vi "Enqueue.vi"(5 "QueName":string="BaseVisQue", 7 "Priority? (F)":bool, 8 "Error":errorcluster[](array[cluster]), 9 "Data":variant, 10 "Message":string) -> (0 "Error":errorcluster[](array[cluster]))   [LabVIEW 2017, in "Visualization.lvlib" / "VisualizeBase_class.lvclass"]
uses:
  VisializeBase_class/VisualizeBase_class.lvclass
  Typedefs/MsgType.ctl
  <userlib>/NIST/NISTErrorLib/NISTErrorLib.lvlib
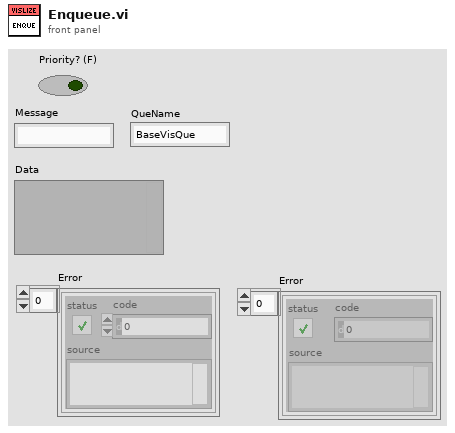
[diagram p1: front panel]
types:
  T1 = typedef "Visualization.lvlib/VisualizeBase_class.lvclass/MsgType.ctl" = cluster{"Message":string, "Data":variant}
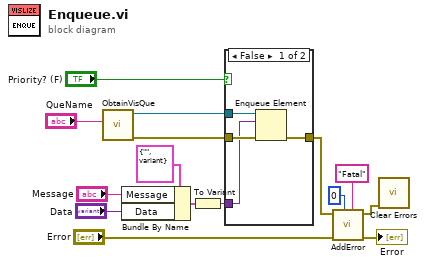
[diagram p0: block diagram]
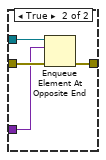
[diagram p2: hidden frame]
diagram:
  n1 = call "ObtainVisQue.vi"("QueName"="QueName") -> ("error out"=w10:errorcluster, "queue out"=w14:refnum<queue>)  [unwired: 9 in]
  n2 = Bundle By Name(cluster=T1 {"Message"="", "Data"=variant} ("clMsgType"), "Message"="Message", "Data"="Data") -> (w9:T1)
  n3 = To Variant(anything=w9) -> (Variant=w8:variant)
  n4 = case shown="False" "Priority? (F)" {
    tunnel: w14 -> [w18 w23]
    tunnel: w10 -> [w19 w22]
    tunnel: w8 -> [w17 w21]
    tunnel: [w16 w20] -> w7
    frame False {
      n5 = Enqueue Element(queue=w18, element=w17, error in (no error)=w19) -> (error out=w16:errorcluster)  [unwired: 1 in, 2 out]
    }
    frame True {
      n6 = Enqueue Element At Opposite End(queue=w23, element=w21, error in (no error)=w22) -> (error out=w20:errorcluster)  [unwired: 1 in, 2 out]
    }
  }
  n7 = call <userlib>:"AddError.vi"("Severity"="Fatal" ("String"), "Priority"=u8 0, "ErrorArray"="Error", "error in (no error)"=w7) -> ("ErrorArray"=→"Error":errorcluster[], "error out"=w2:errorcluster)  [unwired: 6 in]
  n8 = call <vilib>:"Clear Errors.vi"("error in (no error)"=w2) -> ()  [unwired: 5 in, 2 out]
